vi "rad_Open System Config Session.vi"(5 "Password":string, 8 "error in (no error)":errorcluster, 11 "Target settings":T1={"Hostname"="", "Serial number"="", "Product name"="", "Product code"=0, "System status"="", "Credential type"=enum."None/Unlocked", "User added?"=FALSE, "Primary NIC"={"MAC address"="", "IP Address Request Mode"=2, "IP address"="", "Subnet mask"="", "Gateway"="", "DNS server"=""}} {"Primary NIC"."IP Address Request Mode" items=["Static"=1, "DHCP/Link-Local"=2, "Link-Local Only"=4, "DHCP Only"=8]}) -> (0 "error out":errorcluster, 1 "Password out":string, 2 "Cancelled":bool, 3 "Session out":refnum<k21>)   [LabVIEW 2020]
uses:
  <vilib>/nisyscfg/nisyscfg.lvlib
  <vilib>/nisyscfg/Close (System).vi
  rad_Globals.vi
  Targets/TypeDefs/rad_Initialize Access Types.ctl
  Targets/TypeDefs/rad_Target Information.ctl
  Targets/TypeDefs/rad_Target Network Settings.ctl
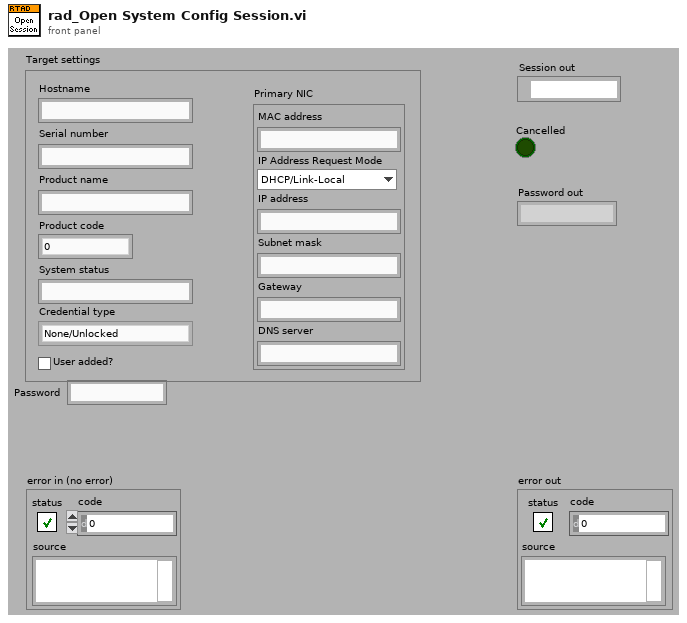
[diagram p1: front panel]
types:
  T1 = typedef "rad_Target Information.ctl" = cluster{"Hostname":string, "Serial number":string, "Product name":string, "Product code":i32, "System status":string, "Credential type":enum16{"None/Unlocked", "FTP Password", "NIAuth Credentials"}, "User added?":bool, "Primary NIC":T2}
  T2 = typedef "rad_Target Network Settings.ctl" = cluster{"MAC address":string, "IP Address Request Mode":i32, "IP address":string, "Subnet mask":string, "Gateway":string, "DNS server":string}
  T3 = typedef "rad_Initialize Access Types.ctl" = enum16{"Anonymous read-only", "Admin unless unlocked", "Admin always"}
  T4 = enum16{"None/Unlocked", "FTP Password", "NIAuth Credentials"}
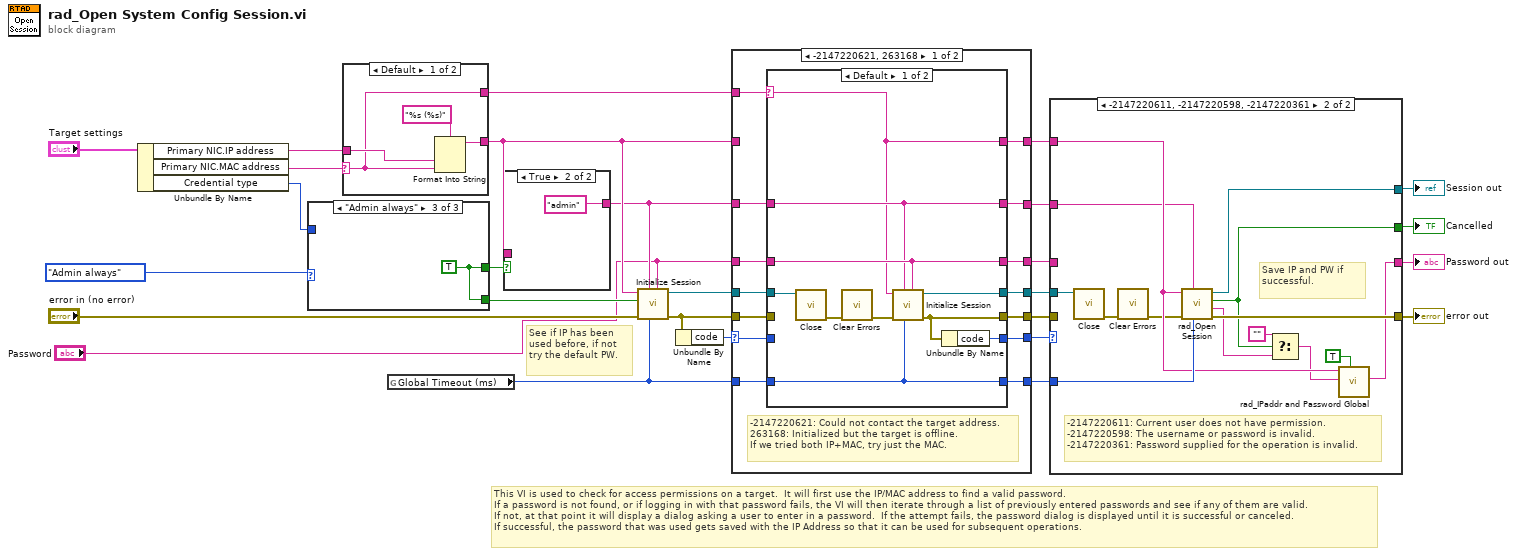
[diagram p0: block diagram]
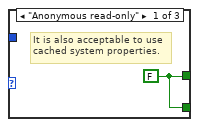
[diagram p4: hidden frame]
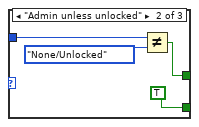
[diagram p5: hidden frame]
diagram:
  # "This VI is used to check for access permissions on a target.  It will first use the IP/MAC address to find a valid password. \nIf a password is not found, or if logging in with that password fails, the VI will then iterate through a list of previously entered passwords and see if any of them are valid.\nIf not, at that point it will display a dialog asking a user to enter in a password.  If the attempt fails, the password dialog is displayed until it is successful or canceled. \nIf successful, the password that was used gets saved with the IP Address so that it can be used for subsequent operations."
  # "See if IP has been used before, if not try the default PW."
  n1 = Unbundle By Name("Target settings") -> ("Primary NIC.IP address"=w20:string, "Primary NIC.MAC address"=w21:string, "Credential type"=w19:T4)
  n2 = case shown="\"Admin always\"" rad_Initialize_Access_Types."Admin always" ("Access requirement (admin unless unlocked)") {
    tunnel: w19 -> [_ w31 _]
    tunnel: [w28 w30 w33] -> w18
    tunnel: [w28 TRUE w33] -> w17
    frame "Anonymous read-only" {
      w28 = FALSE
      # "It is also acceptable to use\ncached system properties."
    }
    frame "Admin unless unlocked" {
      n3 = Not Equal?(x=w31, y=T4."None/Unlocked") -> (x != y?=w30:bool)
    }
    frame "Admin always" {
      w33 = TRUE
    }
  }
  n4 = case shown="Default" w21 {
    selector: w21 -> [w34 _]
    tunnel: w20 -> [w35 w38]
    tunnel: [w36 w38] -> w14
    tunnel: [w34 _] -> w4
    frame Default {
      n5 = Format Into String(format string="%s (%s)", w35, w34) -> (resulting string=w36:string)  [unwired: 2 in, 1 out]
    }
    frame "" {
    }
  }
  n6 = global read "rad_Globals.vi" "Global Timeout (ms)"() -> (w3:u32)
  n7 = case shown="True" w18 {
    tunnel: w14 -> [_ _]
    tunnel: [_ "admin"] -> w12
    frame False {
    }
    frame True {
    }
  }
  n8 = call <vilib>:"Initialize Session.vi"("Password"="Password", "Connect Timeout (4000 ms)"=w3, "User Name"=w12, "error in (no error)"="error in (no error)", "Force Property Refresh (T)"=w17, "Target (localhost)"=w14) -> ("error out"=w7:errorcluster, "Session out"=w9:refnum<k21>)  [unwired: 4 in]
  n9 = Unbundle By Name(w7) -> ("code"=w16:i32)
  n10 = case shown="-2147220621, 263168" w16 {
    selector: w16 -> [w40 w74]
    tunnel: [w48 w74] -> w15
    tunnel: w14 -> [_ w73]
    tunnel: [w42 w73] -> w13
    tunnel: w12 -> [w47 w72]
    tunnel: [w43 w72] -> w11
    tunnel: "Password" -> [w46 w71]
    tunnel: [w44 w71] -> w10
    tunnel: w9 -> [w52 w70]
    tunnel: [w51 w70] -> w8
    tunnel: w7 -> [w50 w69]
    tunnel: [w49 w69] -> w6
    tunnel: w3 -> [w45 w68]
    tunnel: [w41 w68] -> w5
    tunnel: w4 -> [w53 _]
    frame -2147220621, 263168 {
      # "-2147220621: Could not contact the target address.\n263168: Initialized but the target is offline.\nIf we tried both IP+MAC, try just the MAC."
      n11 = case shown="Default" w53 {
        selector: w53 -> [w55 _]
        tunnel: w52 -> [w63 w67]
        tunnel: [w58 w67] -> w51
        tunnel: w50 -> [_ w66]
        tunnel: [w60 w66] -> w49
        tunnel: [w59 w65] -> w48
        tunnel: w47 -> [w56 _]
        tunnel: w46 -> [w57 w64]
        tunnel: w45 -> [w54 _]
        tunnel: [w57 w64] -> w44
        tunnel: [w56 _] -> w43
        tunnel: [w55 _] -> w42
        tunnel: [w54 _] -> w41
        tunnel: w40 -> [_ w65]
        frame Default {
          n12 = call-poly <vilib>:"Close.vi"("Session in"=w63) -> ("error out"=w62:errorcluster)  [unwired: 10 in]
          n13 = call <vilib>:"Clear Errors.vi"("error in (no error)"=w62) -> ("error out"=w61:errorcluster)  [unwired: 5 in, 1 out]
          n14 = call <vilib>:"Initialize Session.vi"("Password"=w57, "Connect Timeout (4000 ms)"=w54, "User Name"=w56, "error in (no error)"=w61, "Target (localhost)"=w55) -> ("error out"=w60:errorcluster, "Session out"=w58:refnum<k21>)  [unwired: 5 in]
          n15 = Unbundle By Name(w60) -> ("code"=w59:i32)
        }
        frame "" {
        }
      }
    }
    frame Default {
    }
  }
  n16 = case shown="-2147220611, -2147220598, -2147220361" w15 {
    tunnel: w6 -> [w77 _]
    tunnel: [w77 w89] -> w27
    tunnel: w8 -> [w76 w91]
    tunnel: [w76 w90] -> w24
    tunnel: w13 -> [_ w87]
    tunnel: [_ w81] -> w26
    tunnel: w5 -> [_ w88]
    tunnel: [w75 w86] -> w23
    tunnel: w10 -> [w75 _]
    tunnel: w11 -> [_ w83]
    frame Default {
    }
    frame -2147220611, -2147220598, -2147220361 {
      # "Save IP and PW if successful."
      # "-2147220611: Current user does not have permission.\n-2147220598: The username or password is invalid.\n-2147220361: Password supplied for the operation is invalid."
      n17 = call-poly <vilib>:"Close.vi"("Session in"=w91) -> ("error out"=w85:errorcluster)  [unwired: 10 in]
      n18 = call <vilib>:"Clear Errors.vi"("error in (no error)"=w85) -> ("error out"=w84:errorcluster)  [unwired: 5 in, 1 out]
      n19 = call "rad_Open Session.vi"("Timeout ms (4s)"=w88, "User name"=w83, "error in (no error)"=w84, "Target Address"=w87) -> ("error out"=w89:errorcluster, "Password Out"=w80:string, "Cancelled"=w81:bool, "session out"=w90:refnum<k21>)  [unwired: 4 in]
      n20 = Select(t="", s=w81, f=w80) -> (s? t:f=w79:string)
      n21 = call "rad_IPaddr and Password Global.vi"("Read(F)/Write(T)"=TRUE, "Password"=w79, "IP/MAC Address"=w87) -> ("Password"=w86:string)  [unwired: 7 in, 1 out]
    }
  }
  "error out" <- w27
  "Session out" <- w24
  "Cancelled" <- w26
  "Password out" <- w23
